vi "Serial Quick Test.vi"() -> ()   [LabVIEW 2017]
uses:
  Serial Device.lvclass
  Simulated Serial Device_class/Simulated Serial Device.lvclass
  C:/LGP5/Resources/Unit-Testing/Serial Project/Libraries/Serial Device_class/Serial Device.lvclass
panel:
  out "Response to Sample Command":string
  in  "Simulate?":bool=TRUE
  in  "error in (no error)":errorcluster
  out "error out":errorcluster
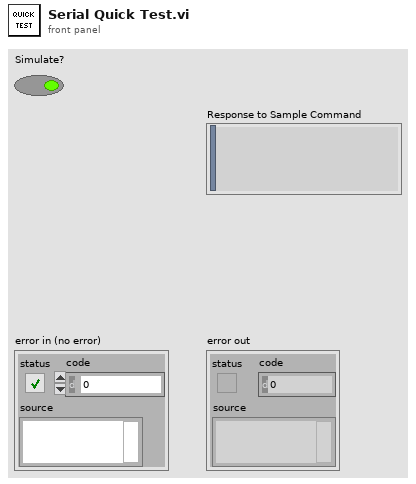
[diagram p1: front panel]
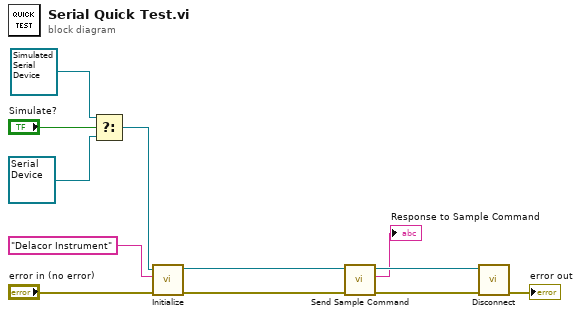
[diagram p0: block diagram]
diagram:
  n1 = Select(t=refnum<class "Simulated Serial Device.lvclass"> refnum ("Simulated Serial Device.lvclass"), s="Simulate?", f=refnum<class "Serial Device.lvclass"> refnum ("Serial Device in")) -> (s? t:f=w7:refnum<class "Serial Device.lvclass">)
  n2 = call-dynamic "Initialize.vi"("error in (no error)"="error in (no error)", "Serial Port"="Delacor Instrument" ("Instrument Name contains"), "Serial Device in"=w7) -> ("error out"=w4:errorcluster, "Serial Device out"=w5:refnum<class "Serial Device.lvclass">)  [unwired: 7 in]
  n3 = call-dynamic "Send Sample Command.vi"("error in (no error)"=w4, "Serial Device"=w5) -> ("error out"=w2:errorcluster, "Response to Sample Command"=→"Response to Sample Command":string, "Serial Device Out"=w3:refnum<class "Serial Device.lvclass">)  [unwired: 7 in]
  n4 = call-dynamic "Disconnect.vi"("error in (no error)"=w2, "Serial Device in"=w3) -> ("error out"=→"error out":errorcluster)  [unwired: 8 in, 1 out]
